vi "FeedBack Chanel.vi"(0 "Test Name":string, 1 "WFGraph Refnum":refnum<vi>, 5 "Channels (Int)":i32[](array[numeric]), 7 "FeedBack Channel":string[](array[string])=["fgdgfvcbc", "vnfhgjkn", "21354682"], 9 "Wait/Poll (ms)":u32, 11 "Parameter":u8) -> (4 "Out":i32, 6 "Array":bool[](array[boolean]), 10 "Fail":bool, 12 "Input Status":bool[](array[boolean]), 13 "Channel No":i32[](array[numeric]))   [LabVIEW 2015]
uses:
  Galobal variable_TI.vi
  Project Setup/Globle Variable/GR_Servo.vi
panel:
  out "Pokayoka Result":cluster{"Sensor Name":string, "Boolean":bool}[](array[cluster])
  out "output array":bool[](array[boolean])
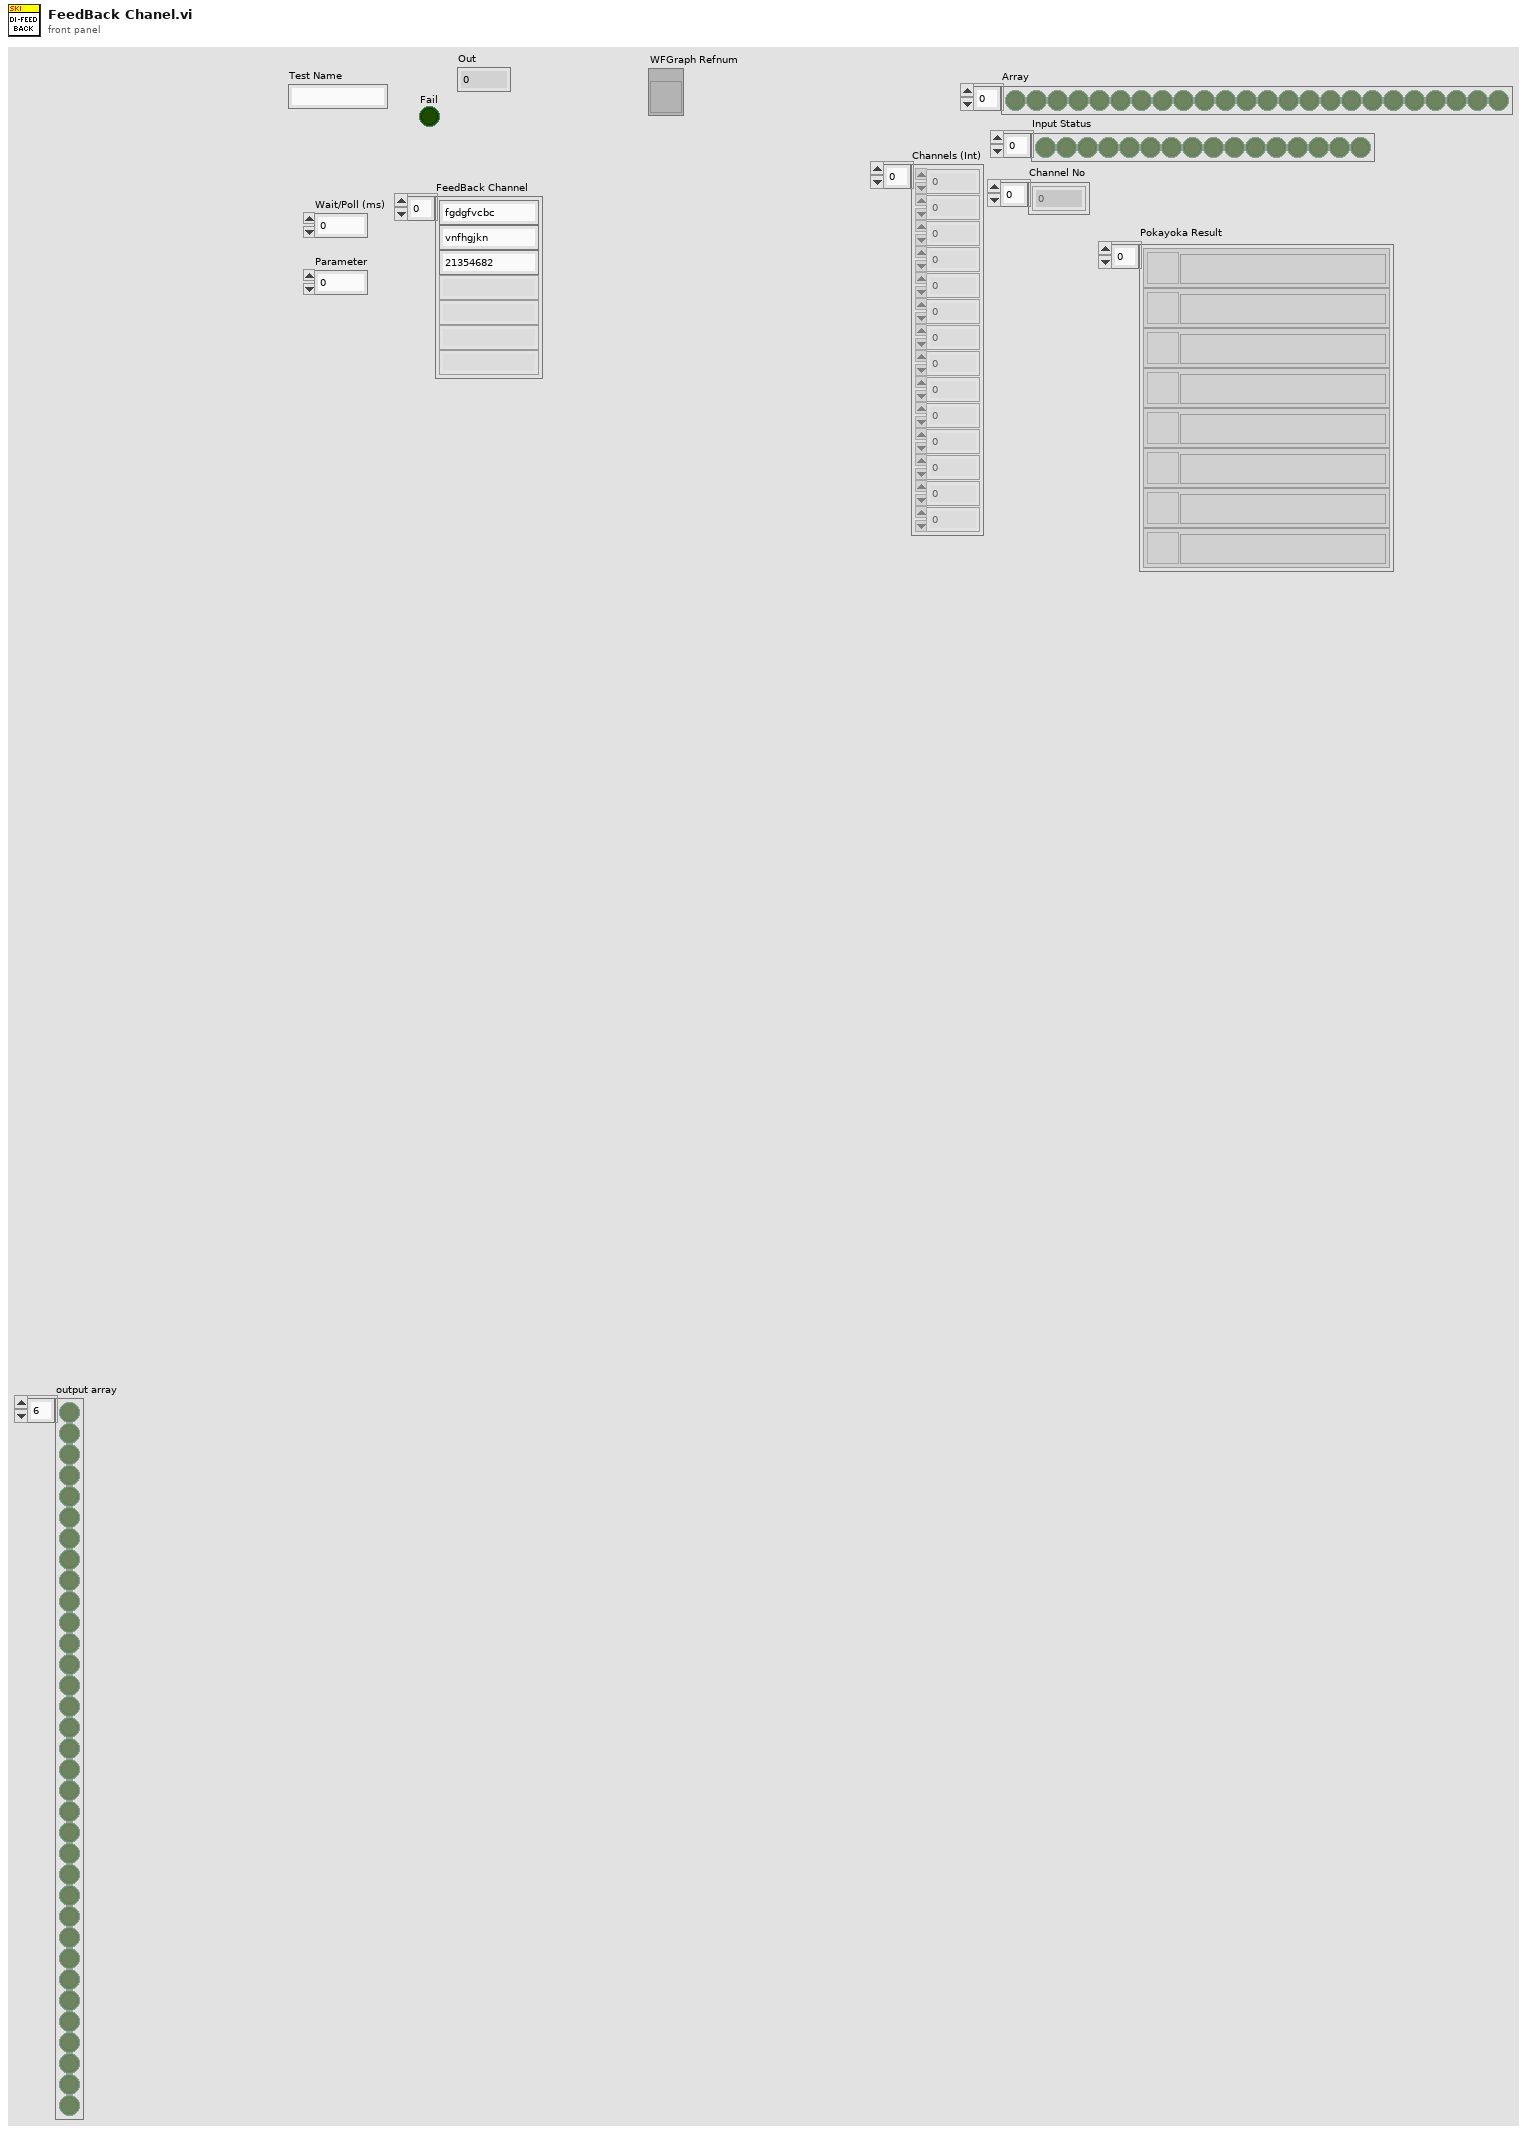
[diagram p1: front panel]
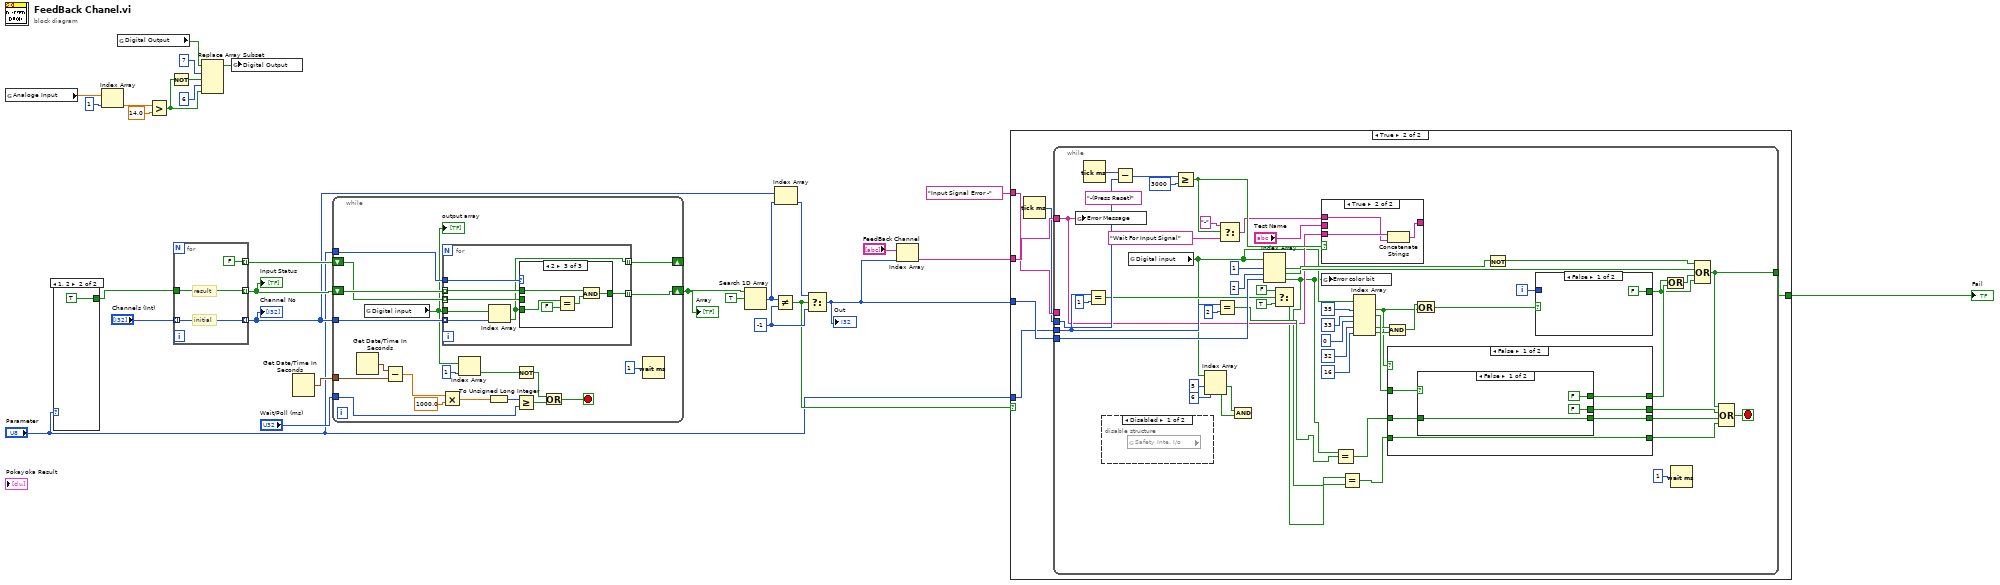
[diagram p0: block diagram]
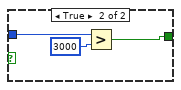
[diagram p4: hidden frame]
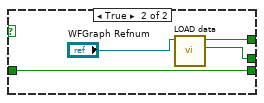
[diagram p5: hidden frame]
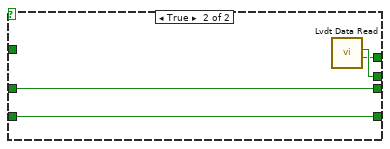
[diagram p6: hidden frame]
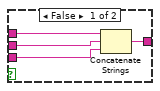
[diagram p7: hidden frame]
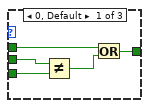
[diagram p8: hidden frame]
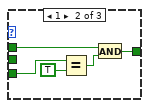
[diagram p9: hidden frame]
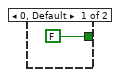
[diagram p10: hidden frame]
diagram:
  w29 = -1 ("y")
  n1 = global read "Galobal variable_TI.vi" "Analoge Input"() -> (w1:dbl[])
  n2 = case shown="1, 2" "Parameter" {
    tunnel: [FALSE TRUE] -> w20
    frame 0, Default {
    }
    frame 1, 2 {
    }
  }
  n3 = Index Array(array=w1, index=1) -> (element=w9:dbl)
  n4 = global read "Galobal variable_TI.vi" "Digital Output"() -> (w3:bool[])
  n5 = Greater?(x=w9, y=14.0) -> (0:w6:bool)
  n6 = Not(x=w6) -> (.not. x?=w7:bool)
  n7 = for {
    tunnel: [w34] -> w15 mode=indexing
    tunnel: w20 -> [w34]
    tunnel: "Channels (Int)" -> [w33] mode=indexing
    tunnel: [w33] -> w14 mode=indexing
    tunnel: [FALSE] -> w24 mode=indexing
    # "result"
    # "initial"
  }
  "Input Status" <- w15
  "Channel No" <- w14
  n8 = Replace Array Subset(array=w3, new element #1=w7, index #1=7 ("index"), new element #2=w6, index #2=6 ("index")) -> (w8:bool[])
  n9 = global write "Galobal variable_TI.vi" "Digital Output"(w8) -> ()
  n10 = Get Date/Time In Seconds() -> (seconds since 1Jan1904=w23:timestamp)
  n11 = while {
    tunnel: "Wait/Poll (ms)" -> [w39]
    tunnel: w23 -> [w53]
    tunnel: w14 -> [w48]
    tunnel: "Parameter" -> [w47]
    shift-right: [w46] -> w26
    shift-left: w15 -> [w44]
    shift-right: [w45] -> _
    shift-left: w24 -> [w43]
    stop <- w41 stop-if-true
    n12 = Get Date/Time In Seconds() -> (seconds since 1Jan1904=w54:timestamp)
    n13 = global read "Galobal variable_TI.vi" "Digital input"() -> (w35:bool[])
    "output array" <- w35
    n14 = Subtract(x=w54, y=w53) -> (x-y=w52:dbl)
    n15 = Multiply(x=w52, y=1000.0) -> (x*y=w50:dbl)
    n16 = for {
      tunnel: w43 -> [w56] mode=indexing
      tunnel: w44 -> [w58] mode=indexing
      tunnel: w35 -> [w61]
      tunnel: w48 -> [w60] mode=indexing
      tunnel: w47 -> [w59]
      tunnel: [w57] -> w46 mode=indexing
      tunnel: [w55] -> w45 mode=indexing
      n17 = Index Array(array=w61, index=w60) -> (element=w55:bool)
      n18 = case shown="2" w59 {
        tunnel: w55 -> [w66 w69 w76]
        tunnel: w58 -> [w64 w68 w73]
        tunnel: [w62 w67 w72] -> w57
        tunnel: w56 -> [w65 _ _]
        frame 0, Default {
          n19 = Not Equal?(x=w65, y=w66) -> (x != y?=w63:bool)
          n20 = Or(x=w64, y=w63) -> (x .or. y?=w62:bool)
        }
        frame 1 {
          n21 = Equal?(x=w69, y=TRUE) -> (x = y?=w70:bool)
          n22 = And(x=w68, y=w70) -> (x .and. y?=w67:bool)
        }
        frame 2 {
          n23 = Equal?(x=w76, y=FALSE) -> (x = y?=w74:bool)
          n24 = And(x=w73, y=w74) -> (x .and. y?=w72:bool)
        }
      }
    }
    n25 = Index Array(array=w35, index=1) -> (element=w37:bool)
    n26 = To Unsigned Long Integer(number=w50) -> (unsigned 32bit integer=w49:u32)
    n27 = Not(x=w37) -> (.not. x?=w38:bool)
    n28 = Greater Or Equal?(x=w49, y=w39) -> (x >= y?=w42:bool)
    n29 = Or(x=w38, y=w42) -> (x .or. y?=w41:bool)
    n30 = Wait (ms)(milliseconds to wait=u32 1) -> ()  [unwired: 1 out]
  }
  "Array" <- w26
  n31 = Search 1D Array(1D array=w26, element=TRUE) -> (index of element=w27:i32)  [unwired: 1 in]
  n32 = Not Equal?(x=w27, y=w29) -> (x != y?=w19:bool)
  n33 = Index Array(array=w14, index=w27) -> (element=w28:i32)
  n34 = Select(t=w28, s=w19, f=w29) -> (s? t:f=w18:i32)
  "Out" <- w18
  n35 = Index Array(array="FeedBack Channel", index=w18) -> (element=w17:string)
  n36 = case shown="True" w19 {
    tunnel: w18 -> [_ w79]
    tunnel: w17 -> [_ w82]
    tunnel: "Input Signal Error -" ("string") -> [_ w81]
    tunnel: "Parameter" -> [_ w78]
    tunnel: [_ w77] -> w11
    frame False {
    }
    frame True {
      n37 = Tick Count (ms)() -> (millisecond timer value=w80:u32)
      n38 = while {
        tunnel: w82 -> [w91]
        tunnel: w81 -> [_]
        tunnel: w80 -> [w133]
        tunnel: w79 -> [w120]
        tunnel: w78 -> [w108]
        tunnel: [w110] -> w77
        i -> [w97]
        stop <- w121 stop-if-true
        (unwired) "-(Press Reset)" ("f")
        n39 = global write "GR_Servo.vi" "Error Message"(w91) -> ()
        n40 = Tick Count (ms)() -> (millisecond timer value=w134:u32)
        n41 = Equal?(x=w108, y=u8 1) -> (x = y?=w104:bool)
        n42 = disable-structure shown="Disabled" {
          frame Disabled {
            n43 = global read "Galobal variable_TI.vi" "Safety Inte. I/o"() -> ()  [unwired: 1 out]
          }
          frame Enabled {
          }
        }
        n44 = Subtract(x=w134, y=w133) -> (x-y=w132:u32)
        n45 = global read "Galobal variable_TI.vi" "Digital input"() -> (w90:bool[])
        n46 = Greater Or Equal?(x=w132, y=u32 3000) -> (x >= y?=w130:bool)
        n47 = Index Array(array=w90, index #1=5 ("index"), index #2=6 ("index")) -> (element #1=w87:bool, element #2=w86:bool)
        n48 = Equal?(x=w108, y=u8 2) -> (x = y?=w118:bool)
        n49 = Select(t="-" ("f"), s=w130, f="Wait For Input Signal") -> (s? t:f=w129:string)
        n50 = And(x=w87, y=w86) -> ()  [unwired: 1 out]
        n51 = Index Array(array=w90, index #1=1 ("index"), index #2=2 ("index"), index #3=w120) -> (element #1=w125:bool, element #2=w122:bool, element #3=w84:bool)
        n52 = Select(t=FALSE, s=w104, f=TRUE) -> (s? t:f=w85:bool)
        n53 = case shown="True" w130 {
          tunnel: w91 -> [w160 w163]
          tunnel: "Test Name" -> [w159 _]
          tunnel: w129 -> [w158 w162]
          tunnel: [w157 w161] -> _
          frame False {
            n54 = Concatenate Strings(w158, w159, w160) -> (w157:string)
          }
          frame True {
            n55 = Concatenate Strings(w163, w162) -> (w161:string)
          }
        }
        n56 = global write "Galobal variable_TI.vi" "Error color bit"(w84) -> ()
        n57 = Equal?(x=w84, y=w118) -> (x = y?=w114:bool)
        n58 = Equal?(x=w84, y=w85) -> (x = y?=w83:bool)
        n59 = Index Array(array=w90, index #1=35 ("index"), index #2=33 ("index"), index #3=0 ("index"), index #4=32 ("index"), index #5=16 ("index")) -> (element #1=w95:bool, element #2=w111:bool, element #4=w99:bool, element #5=w98:bool)  [unwired: 1 out]
        n60 = case shown="False" w95 {
          tunnel: w114 -> [w143 w154]
          tunnel: [w145 w156] -> w113
          tunnel: [w144 w155] -> w112
          tunnel: [w142 w154] -> w107
          tunnel: w111 -> [w141 _]
          tunnel: [w140 w153] -> w106
          tunnel: w83 -> [w140 w153]
          frame False {
            n61 = case shown="False" w141 {
              tunnel: [FALSE ("ok") w152] -> w145
              tunnel: [FALSE ("ng") w151] -> w144
              tunnel: [w146 w150] -> w142
              tunnel: w143 -> [w146 w150]
              frame False {
              }
              frame True {
                n62 = call "LOAD data.vi"("WFGraph Refnum"="WFGraph Refnum") -> ("ok"=w152:bool, "ng"=w151:bool)  [unwired: 9 in]
              }
            }
          }
          frame True {
            n63 = call "Lvdt Data Read.vi"() -> ("ng"=w155:bool, "ok"=w156:bool)  [unwired: 10 in]
          }
        }
        n64 = Compound Arithmetic op=AND(w99, w98) -> (w96:bool)
        n65 = Compound Arithmetic op=OR(w96, w95) -> (w94:bool)
        n66 = Not(x=w125) -> (.not. x?=w123:bool)
        n67 = case shown="False" w94 {
          tunnel: w97 -> [_ w139]
          tunnel: [FALSE w137] -> w92
          frame False {
          }
          frame True {
            n68 = Greater?(x=w139, y=3000) -> (0:w137:bool)
          }
        }
        n69 = Compound Arithmetic op=OR(w92, w112) -> (w93:bool)
        n70 = Wait (ms)(milliseconds to wait=u32 1) -> ()  [unwired: 1 out]
        n71 = Compound Arithmetic op=OR(w123, w122, w93, w92) -> (w110:bool)
        n72 = Compound Arithmetic op=OR(w110, w113, w107, w106) -> (w121:bool)
      }
    }
  }
  "Fail" <- w11
